vi "VMI_test_queueing.vi"() -> ()   [LabVIEW 2015]
uses:
  <vilib>/vision/Image Controls.llb/IMAQ Image.ctl
  <vilib>/Platform/TimedLoop/XDataNode/timing_clust.ctl
  <vilib>/Platform/TimedLoop/XDataNode/nitl_modes.ctl
  <vilib>/Platform/TimedLoop/XDataNode/wakeup.ctl
  <vilib>/platform/TimedLoop/XDataNode/XDataNode.xnode
  <vilib>/Platform/TimedLoop/XDataNode/XDNodeRunTimeDep.lvlib
panel:
  out "Display loops":i32[](array[numeric])
  out "Timed loops":i32[](array[numeric])
  out "Number anl\nlops":i32[](array[numeric])
  in  "Boolean 2":bool=TRUE
  in  "Boolean":bool
  in  "Peak Find Settings":T1={"Objects"=0, "Threshold"=128, "Reject Border"=FALSE, "Fill Holes"=FALSE, "Min Object Size"=FALSE, "Min Size"=3, "Max Object Size"=FALSE, "Max Size"=100, "Show Search Area"=FALSE, "Show Center"=TRUE, "Show Bounding Box"=TRUE} {"Objects" items=["Bright Objects", "Dark Objects"]; "Threshold" min=1 max=999999999 step=1; "Max Size" min=1 max=999999999 step=1; "Min Size" min=1 max=999999999 step=1}
  out "Number Points":i32[](array[numeric])
  in  "Total Acquires":i32=1
  in  "Acquire Time":i32
  out "Current Image 2":T2(plugin-control)
  in  "Image Type":T3 items=["Grayscale (U8)", "Grayscale (I16)", "Grayscale (SGL)", "Complex (CSG)", "RGB (U32)", "HSL (U32)", "RGB (U64)", "Grayscale (U16)"]
  in  "File Path":path=path "C:/Users/Parkes/Documents/GitHub/Camera-Acquire_Labview/mcp_hit_test.png"
  out "Error Out":errorcluster
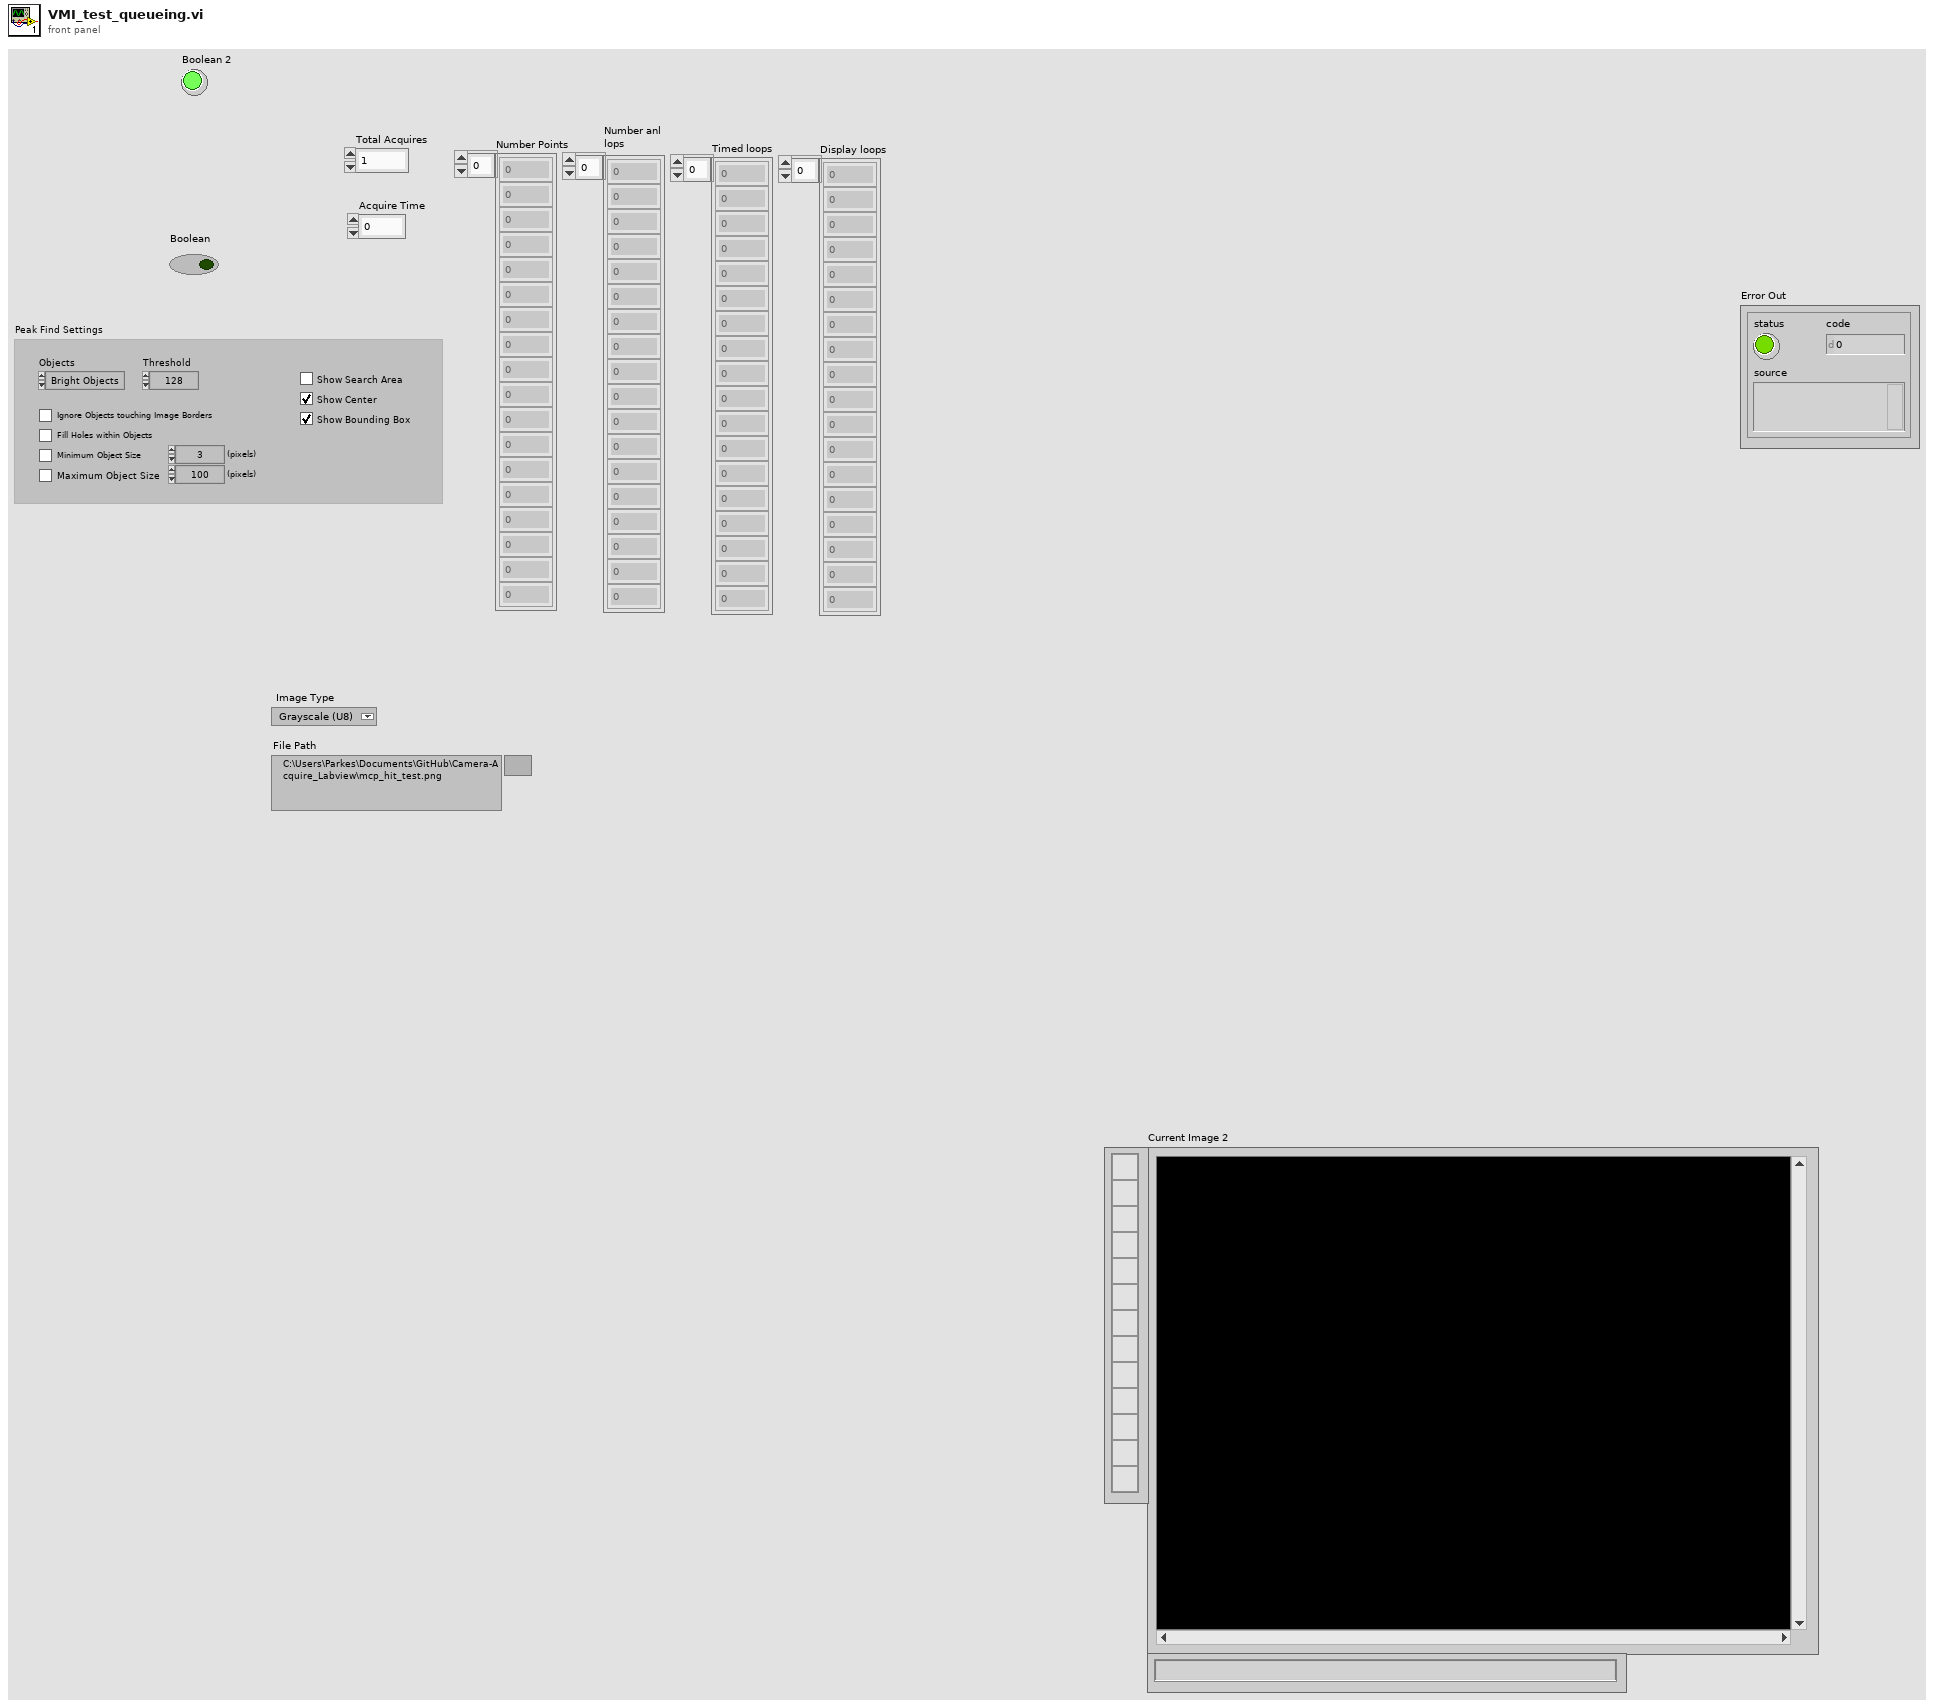
[diagram p1: front panel]
types:
  T1 = cluster{"Objects":u16, "Threshold":i32, "Reject Border":bool, "Fill Holes":bool, "Min Object Size":bool, "Min Size":i32, "Max Object Size":bool, "Max Size":i32, "Show Search Area":bool, "Show Center":bool, "Show Bounding Box":bool}
  T2 = typedef "IMAQ Image.ctl" = refnum<image>
  T3 = typedef "Image Type" = u32
  T4 = typedef "Queue RefNum" = refnum<k1>
  T5 = typedef "XDNodeRunTimeDep.lvlib/timing_clust.ctl" = cluster{"Expected End [f-1]":u64, "Actual End [f-1]":u64, "Finished Late? [f-1]":bool, "Expected End [i-1]":u64, "Actual End [i-1]":u64, "Finished Late? [i-1]":bool, "Expected Start [i]":u64, "Actual Start [i]":u64, "Expected Start [f]":u64, "Actual Start [f]":u64, "Source Name":string, "Structure Name":string, "Period":i64, "Deadline":i64, "Offset":i64, "Start":i64, "Priority":i32, "Timeout":i32, "Mode":T6, "Wakeup Reason":T7, "Error":errorcluster, "Source Type":string, "Secondary Source Type":string, "Global End Time":u64, "Global Start Time":u64, "Frame Duration":u64, "Iteration Duration":u64, "Assigned CPU":i32, "I/O Scan Engine Mode":u32}
  T6 = typedef "XDNodeRunTimeDep.lvlib/nitl_modes.ctl" = enum32{"No Change", "Process missed periods, maintain original phase", "Discard missed periods, maintain original phase", "Process missed periods, ignore original phase", "Discard missed periods, ignore original phase"}
  T7 = typedef "XDNodeRunTimeDep.lvlib/wakeup.ctl" = enum32{"Normal", "Aborted", "Asynchronous wakeup", "Timing source error", "Timed loop error", "Timeout"}
  T8 = cluster{"Object Center":cluster{"X":sgl, "Y":sgl}, "Bounding Box":cluster{"X Left":i32, "Y Top":i32, "X Right":i32, "Y Bottom":i32}, "Area":sgl, "Orientation":sgl, "Aspect Ratio":sgl, "Nb Holes":i32}[]
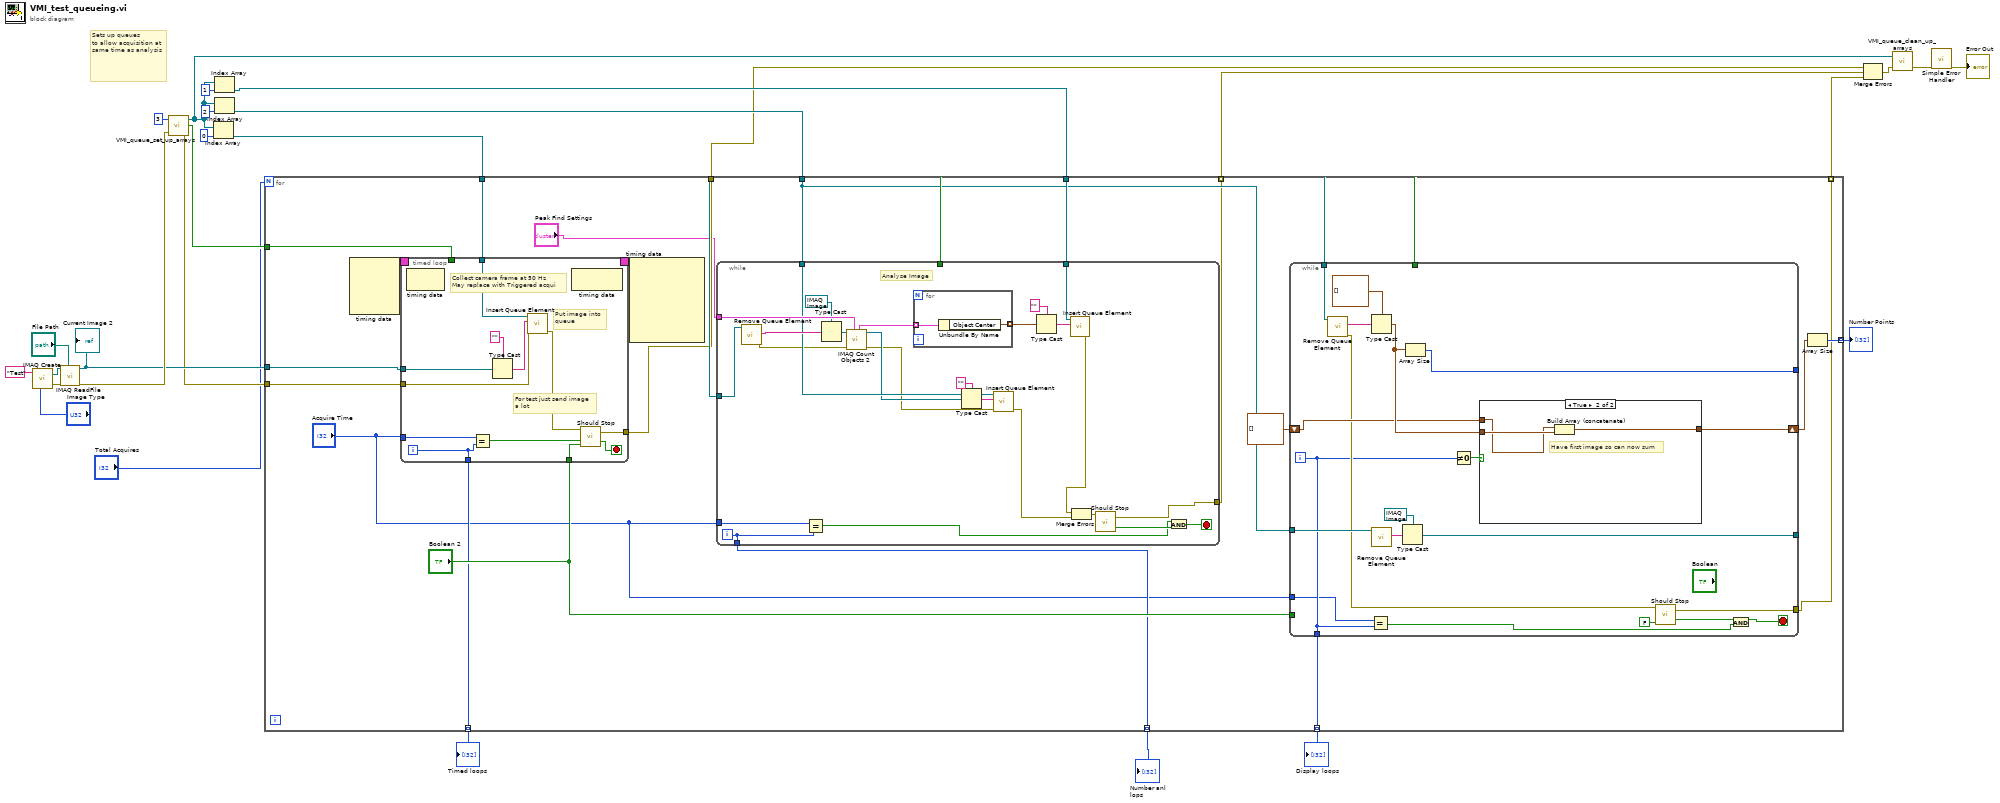
[diagram p0: block diagram]
diagram:
  # "Sets up queues\nto allow acquisition at same time as analysis"
  n1 = call "IMAQ Create"("Image Name"="Test", "Image Type"="Image Type") -> ("New Image"=w19:T2, "error out"=w17:errorcluster)  [unwired: 3 in]
  n2 = call "IMAQ ReadFile"("File Path"="File Path", "error in (no error)"=w17, "Image"=w19) -> ("error out"=w16:errorcluster, "Image Out"=w15:T2)  [unwired: 4 in, 3 out]
  "Current Image 2" <- w15
  n3 = call "VMI_queue_set_up_arrays.vi"("error in (no error)"=w16, "Number of Queues"=3) -> ("error out"=w14:errorcluster, "Stop"=w11:bool, "Queue Array"=w22:T4[])  [unwired: 1 in]
  n4 = Index Array(array=w22, index=0) -> (element=w13:T4)
  n5 = Index Array(array=w22, index=1) -> (element=w12:T4)
  n6 = Index Array(array=w22, index=2) -> (element=w10:T4)
  n7 = for {
    N: "Total Acquires" -> [_]
    tunnel: w15 -> [w46]
    tunnel: w14 -> [w45]
    tunnel: w13 -> [w44]
    tunnel: w12 -> [w43]
    tunnel: w11 -> [w42]
    tunnel: w10 -> [w41]
    tunnel: [w39] -> w8 mode=indexing
    tunnel: [w38] -> w7
    tunnel: [w37] -> w5 mode=indexing
    tunnel: [w36] -> w4 mode=indexing
    tunnel: [w31] -> w3 mode=indexing
    tunnel: [w32] -> w2 mode=indexing
    tunnel: [w30] -> w1 mode=indexing
    n8 = node-c288() -> (w48:T5)  [unwired: 4 in]
    n9 = timed-loop {
      timing: w48 -> [_]
      timing-out: [_] -> w47
      tunnel: w44 -> [w111]
      tunnel: [w109] -> w38
      tunnel: w45 -> [w105]
      tunnel: w46 -> [w108]
      tunnel: "Boolean 2" -> [w104]
      tunnel: "Acquire Time" -> [w103]
      tunnel: w42 -> [_]
      tunnel: [w100] -> w32
      i -> [w100]
      stop <- w101 stop-if-true
      # "Put image into\nqueue"
      # "For test just send image\na lot"
      # "Collect camera frame at 50 Hz\nMay replace with Triggered acqui"
      n10 = node-c288() -> ()  [unwired: 1 in, 1 out]
      n11 = Equal?(x=w103, y=w100) -> (x = y?=w102:bool)
      n12 = Type Cast(type="", x=w108) -> (*(type *) &x=w106:string)
      n13 = call <vilib>:"Insert Queue Element.vi"("error in (no error)"=w105, "queue element"=w106, "queue"=w111) -> ("error out"=w110:errorcluster)  [unwired: 4 in, 2 out]
      n14 = node-c288() -> ()  [unwired: 1 in, 1 out]
      n15 = call "Should Stop.vi"("error in 1"=w110, "Stop Button"=w102, "Look at Stop Button"=w104) -> ("error out"=w109:errorcluster, "Stop"=w101:bool)  [unwired: 2 in]
    }
    n16 = node-c288(w47) -> ()  [unwired: 7 out]
    n17 = while {
      tunnel: w44 -> [w80]
      tunnel: "Peak Find Settings" -> [w95]
      tunnel: w43 -> [w91]
      tunnel: w41 -> [w89]
      tunnel: [w73] -> w37
      tunnel: w42 -> [_]
      tunnel: [w76] -> w31
      tunnel: "Acquire Time" -> [w75]
      i -> [w76]
      stop <- w77 stop-if-true
      # "Analyse Image"
      n18 = call <vilib>:"Remove Queue Element.vi"("queue"=w80) -> ("error out"=w84:errorcluster, "queue element"=w97:string)  [unwired: 5 in, 2 out]
      n19 = Equal?(x=w75, y=w76) -> (x = y?=w74:bool)
      n20 = Type Cast(type=T2 refnum ("Image Out"), x=w97) -> (*(type *) &x=w96:T2)
      n21 = call "IMAQ Count Objects 2"("Settings"=w95, "error in (no error)"=w84, "Image"=w96) -> ("error out"=w83:errorcluster, "Image Out"=w85:T2, "Objects"=w94:T8)  [unwired: 4 in, 2 out]
      n22 = for {
        tunnel: w94 -> [w99] mode=indexing
        tunnel: [w98] -> w90 mode=indexing
        n23 = Unbundle By Name(w99) -> ("Object Center"=w98:cluster{"X":sgl, "Y":sgl})
      }
      n24 = Type Cast(type="", x=w85) -> (*(type *) &x=w87:string)
      n25 = call <vilib>:"Insert Queue Element.vi"("error in (no error)"=w83, "queue element"=w87, "queue"=w89) -> ("error out"=w81:errorcluster)  [unwired: 4 in, 2 out]
      n26 = Type Cast(type="", x=w90) -> (*(type *) &x=w92:string)
      n27 = call <vilib>:"Insert Queue Element.vi"("queue element"=w92, "queue"=w91) -> ("error out"=w79:errorcluster)  [unwired: 5 in, 2 out]
      n28 = Merge Errors(w79, w81) -> (w82:errorcluster)
      n29 = call "Should Stop.vi"("error in 1"=w82) -> ("error out"=w73:errorcluster, "Stop"=w78:bool)  [unwired: 4 in]
      n30 = And(x=w74, y=w78) -> (x .and. y?=w77:bool)
    }
    n31 = while {
      tunnel: w43 -> [w68]
      tunnel: [w52] -> w30
      tunnel: w41 -> [w64]
      shift-right: [w59] -> w40
      shift-left: cluster{"X":sgl, "Y":sgl}[] [] -> [w58]
      tunnel: [w57] -> w36
      tunnel: [w54] -> _
      tunnel: [w56] -> _
      tunnel: w42 -> [_]
      tunnel: "Boolean 2" -> [_]
      tunnel: "Acquire Time" -> [w51]
      i -> [w52]
      stop <- w50 stop-if-true
      n32 = call <vilib>:"Remove Queue Element.vi"("queue"=w68) -> ("error out"=w55:errorcluster, "queue element"=w66:string)  [unwired: 5 in, 2 out]
      n33 = Equal?(x=w51, y=w52) -> (x = y?=w49:bool)
      n34 = Type Cast(type=cluster{"X":sgl, "Y":sgl}[] [], x=w66) -> (*(type *) &x=w60:cluster{"X":sgl, "Y":sgl}[])
      n35 = call <vilib>:"Remove Queue Element.vi"("queue"=w64) -> ("queue element"=w63:string)  [unwired: 5 in, 3 out]
      n36 = Type Cast(type=T2 refnum ("Image Out"), x=w63) -> (*(type *) &x=w54:T2)
      n37 = Array Size(array=w60) -> (size(s)=w56:i32)
      n38 = Not Equal To 0?(x=w52) -> (x != 0?=w61:bool)
      n39 = case shown="True" w61 {
        tunnel: w60 -> [w69 w72]
        tunnel: [w69 w70] -> w59
        tunnel: w58 -> [_ w71]
        frame False {
          # "Nothing exisiting so clear"
        }
        frame True {
          # "Have first image so can now sum"
          n40 = Build Array (concatenate)(w71, w72) -> (w70:cluster{"X":sgl, "Y":sgl}[])
        }
      }
      n41 = call "Should Stop.vi"("error in 1"=w55, "Look at Stop Button"=FALSE) -> ("error out"=w57:errorcluster, "Stop"=w67:bool)  [unwired: 3 in]
      n42 = And(x=w67, y=w49) -> (x .and. y?=w50:bool)
    }
    n43 = Array Size(array=w40) -> (size(s)=w39:i32)
  }
  "Number Points" <- w8
  "Number anl\nlops" <- w3
  "Timed loops" <- w2
  "Display loops" <- w1
  n44 = Merge Errors(w7, w5, w4) -> (w6:errorcluster)
  n45 = call "VMI_queue_clean_up_arrays.vi"("error in (no error)"=w6, "Queue Array"=w22) -> ("error out"=w24:errorcluster)  [unwired: 1 in]
  n46 = call <vilib>:"Simple Error Handler.vi"("error in (no error)"=w24) -> ("error out"=→"Error Out":errorcluster)  [unwired: 4 in, 4 out]
